vi "Subtract (Elementwise) - RM,R.vi"(1 "Real Scalar c":dbl, 2 "Real Matrix A":T1) -> (0 "A - c":T1)   [LabVIEW 2017, in "NI_Matrix.lvlib"]
doc: "Computes the difference of the inputs."
uses:
  NI_Matrix.lvlib
  RealMatrix.ctl
  Array To Matrix - RA2.vi
  Matrix To Array - RM.vi
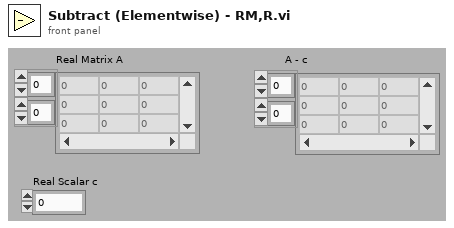
[diagram p1: front panel]
types:
  T1 = typedef "NI_Matrix.lvlib/RealMatrix.ctl" = dbl[][]
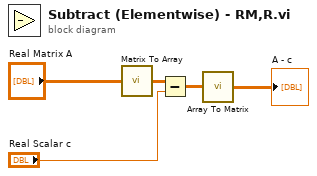
[diagram p0: block diagram]
diagram:
  n1 = call-poly "Matrix To Array.vi"("Real Matrix"="Real Matrix A") -> ("Real 2D Array"=w4:dbl[][])
  n2 = Subtract(x=w4, y="Real Scalar c") -> (x-y=w2:dbl[][])
  n3 = call-poly "Array To Matrix.vi"("Real 2D Array"=w2) -> ("Real Matrix"=→"A - c":T1)
